vi "BK Precision 178XB Monitor Output.vi"() -> ()   [LabVIEW 2019]
doc: "This example VI monitors the output voltage and current from the power supply."
uses:
  BK Precision 178XB Series.lvlib
panel:
  out "Temperature":dbl
  in  "Update Time (1000)":u16=1000 min=1000 step=1
  out "Current":dbl format="%#.2g"
  out "Voltage":dbl format="%#.2g"
  in  "Current Limit (0)":dbl min=0.0 max=6.0 format="%#.2g"
  in  "Output Voltage (0)":dbl min=0.0 max=18.0 format="%#.2g"
  in  "Maximum Output Voltage (18)":dbl=18.0 min=0.0 max=72.0 format="%#.2g"
  in  "VISA resource name":refnum<visa-resource-name>
  in  "stop":bool
  # "Instructions:  Setup the values for max output voltage, output voltage, and current limit.  Update time configures how often display values should be read for monitoring."
  # "(c) 2009 B&K PRECISION CORPORATION.  ALL RIGHTS RESERVED."
  # "ms"
  # "A"
  # "V"
  # "A"
  # "V"
  # "V"
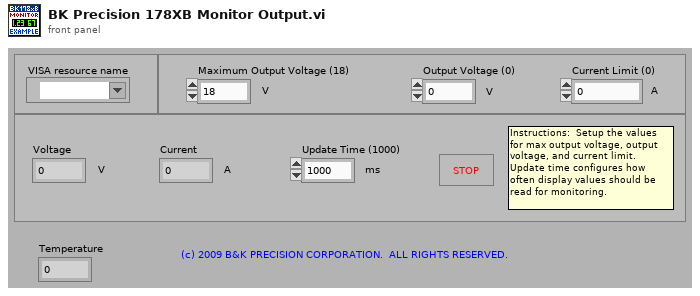
[diagram p1: front panel]
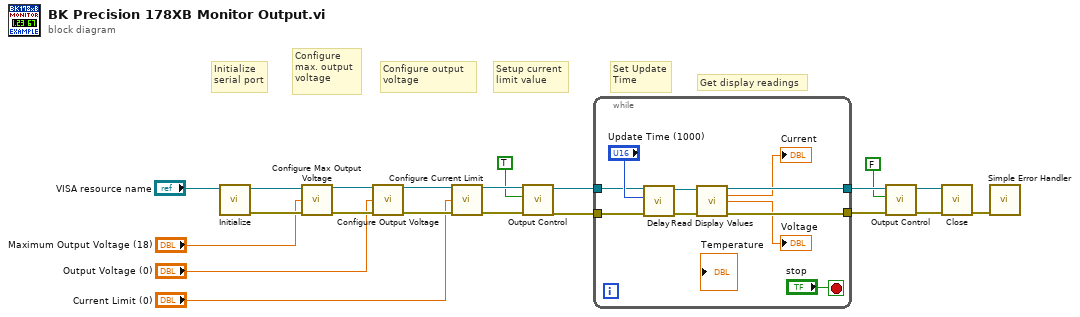
[diagram p0: block diagram]
diagram:
  # "Setup current\nlimit value"
  # "Configure output\nvoltage"
  # "Configure\nmax. output\nvoltage"
  # "Initialize\nserial port"
  # "Get display readings"
  # "Set Update\nTime"
  n1 = call "Initialize.vi"("VISA resource name"="VISA resource name") -> ("error out"=w19:errorcluster, "VISA resource name out"=w20:refnum<visa-resource-name>)  [unwired: 9 in]
  n2 = call "Configure Max Output Voltage.vi"("VISA resource name"=w20, "Maximum Output Voltage (18)"="Maximum Output Voltage (18)", "error in (no error)"=w19) -> ("VISA resource name out"=w18:refnum<visa-resource-name>, "error out"=w15:errorcluster)  [unwired: 11 in]
  n3 = call "Configure Output Voltage.vi"("VISA resource name"=w18, "Output Voltage (0)"="Output Voltage (0)", "error in (no error)"=w15) -> ("VISA resource name out"=w17:refnum<visa-resource-name>, "error out"=w16:errorcluster)  [unwired: 11 in]
  n4 = call "Configure Current Limit.vi"("VISA resource name"=w17, "Current Limit (0)"="Current Limit (0)", "error in (no error)"=w16) -> ("VISA resource name out"=w14:refnum<visa-resource-name>, "error out"=w13:errorcluster)  [unwired: 11 in]
  n5 = call "Output Control.vi"("error in (no error)"=w13, "Enable Output Terminals (F: Off)"=TRUE, "VISA resource name"=w14) -> ("error out"=w6:errorcluster, "VISA resource name out"=w7:refnum<visa-resource-name>)  [unwired: 7 in]
  n6 = while {
    tunnel: [w25] -> w4
    tunnel: [w24] -> w5
    tunnel: w7 -> [w27]
    tunnel: w6 -> [w26]
    stop <- "stop" stop-if-true
    n7 = call "Delay.vi"("error in (no error)"=w26, "Delay Value (100)"="Update Time (1000)", "VISA resource name"=w27) -> ("error out"=w28:errorcluster, "VISA resource name out"=w29:refnum<visa-resource-name>)  [unwired: 7 in]
    n8 = call "Read Display Values.vi"("VISA resource name"=w29, "error in (no error)"=w28) -> ("VISA resource name out"=w25:refnum<visa-resource-name>, "Terminal Output Current"=→"Current":dbl, "Terminal Output Voltage"=→"Voltage":dbl, "error out"=w24:errorcluster)  [unwired: 10 in]
  }
  n9 = call "Output Control.vi"("error in (no error)"=w5, "Enable Output Terminals (F: Off)"=FALSE, "VISA resource name"=w4) -> ("error out"=w2:errorcluster, "VISA resource name out"=w3:refnum<visa-resource-name>)  [unwired: 7 in]
  n10 = call "Close.vi"("error in (no error)"=w2, "VISA resource name"=w3) -> ("error out"=w21:errorcluster)  [unwired: 9 in]
  n11 = call <vilib>:"Simple Error Handler.vi"("error in (no error)"=w21) -> ()  [unwired: 4 in, 5 out]
